vi "Analysis.vi"(8 "error in (no error)":errorcluster, 11 "Elevator Controller in":refnum<class "Elevator Controller.lvclass">) -> (0 "error out":errorcluster, 3 "Elevator Controller out":refnum<class "Elevator Controller.lvclass">)   [LabVIEW 2019, in "Elevator Controller.lvlib" / "Elevator Controller.lvclass"]
uses:
  Elevator Controller.lvclass
  State -Enum.ctl
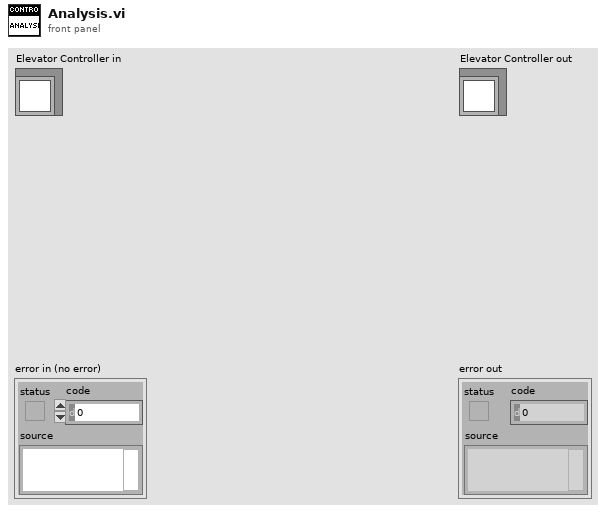
[diagram p1: front panel]
types:
  T1 = typedef "Elevator Controller.lvlib/Elevator Controller.lvclass/State -Enum.ctl" = enum16{"Initial", "Wait for First Request", "Start and Move", "Analysis", "Continue Travel", "Stop at Floor", "Open and Close Door Sequence", "No request Remaining", "Emergency Call", "Terminate Process"}
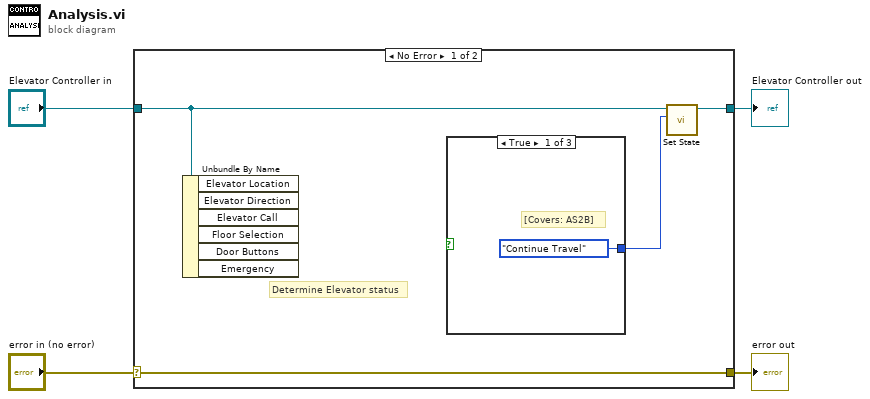
[diagram p0: block diagram]
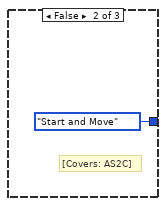
[diagram p2: hidden frame]
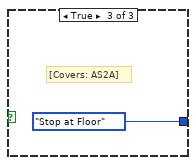
[diagram p3: hidden frame]
diagram:
  n1 = case shown="No Error" "error in (no error)" {
    selector: "error in (no error)" -> [w8 w13]
    tunnel: [w8 w13] -> w3
    tunnel: [w6 w12] -> w1
    tunnel: "Elevator Controller in" -> [w7 w12]
    frame No Error {
      # "Determine Elevator status"
      n2 = Unbundle By Name(w7) -> ()  [unwired: 6 out]
      n3 = case shown="\"Continue in the current direction\"" {
        selector: _ -> [_ _ _]
        tunnel: [State_-Enum."Continue Travel" ("State") State_-Enum."Start and Move" ("State") State_-Enum."Stop at Floor" ("State")] -> w5
        frame True {
          # "[Covers: AS2B]"
        }
        frame False {
          # "[Covers: AS2C]"
        }
        frame True {
          # "[Covers: AS2A]"
        }
      }
      n4 = call "Set State.vi"("State"=w5, "Elevator Controller in"=w7) -> ("Elevator Controller out"=w6:refnum<class "Elevator Controller.lvclass">)  [unwired: 8 in, 1 out]
    }
    frame Error {
    }
  }
  "error out" <- w3
  "Elevator Controller out" <- w1
